vi "temp_logger.vi"() -> ()   [LabVIEW 2017]
panel:
  in  "stop":bool
  out "time":string
  out "Thermometer":dbl(slide) scale=-25.0..60.0
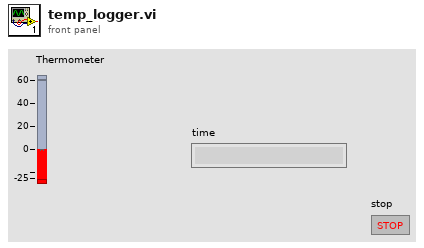
[diagram p1: front panel]
types:
  T1 = typedef "LVDateTimeRec.ctl" = cluster{"fractional second":dbl, "second":i32, "minute":i32, "hour":i32, "day of month":i32, "month":i32, "year":i32, "day of week":i32, "day of year":i32, "DST":i32}
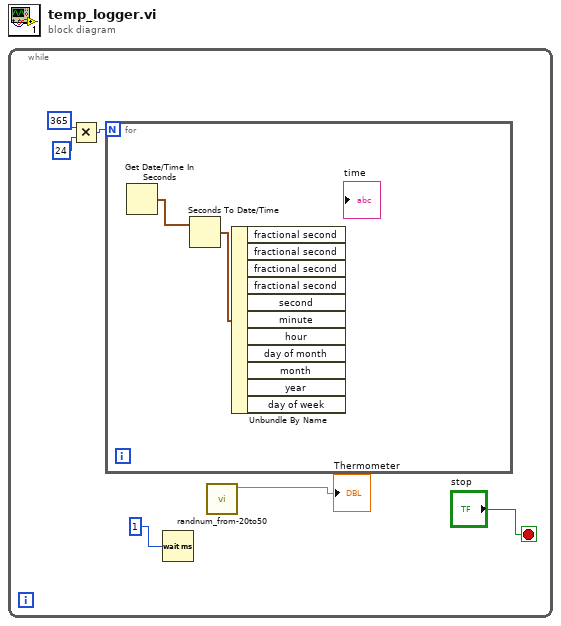
[diagram p0: block diagram]
diagram:
  n1 = while {
    stop <- "stop" stop-if-true
    n2 = Multiply(x=365, y=24) -> (x*y=w3:i32)
    n3 = for {
      N: w3 -> [_]
      n4 = Get Date/Time In Seconds() -> (seconds since 1Jan1904=w8:timestamp)
      n5 = Seconds To Date/Time(time stamp (now)=w8) -> (date time rec=w7:T1)  [unwired: 1 in]
      n6 = Unbundle By Name(w7) -> ()  [unwired: 11 out]
    }
    n7 = Wait (ms)(milliseconds to wait=1) -> ()  [unwired: 1 out]
    n8 = call "randnum_from-20to50.vi"() -> ("Numeric"=→"Thermometer":dbl)  [unwired: 11 in]
  }
